vi "GetCalInfo.vi"(6 "Legacy (f)?":bool, 8 "error in (no error)":errorcluster) -> (0 "error out":errorcluster, 2 "CalInfo":T1)   [LabVIEW 2011]
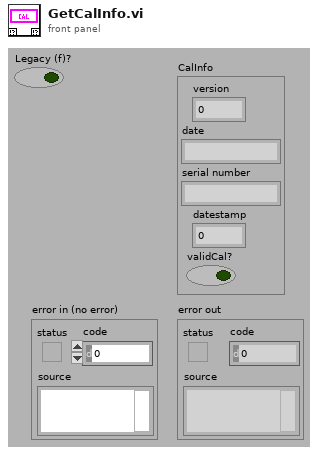
[diagram p1: front panel]
types:
  T1 = cluster{"version":u8, "date":string, "serial number":string, "datestamp":dbl, "validCal?":bool}
  T2 = cluster{"Command":string, "appended array":variant[]}
  T3 = cluster{"Command":string, "appended array":variant[]}[]
  T4 = cluster{"version":u8, "date":string, "serial number":string}
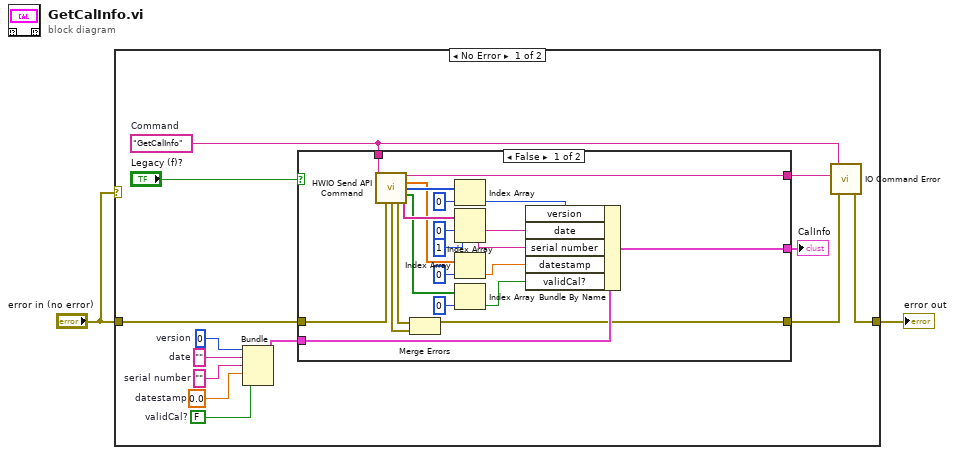
[diagram p0: block diagram]
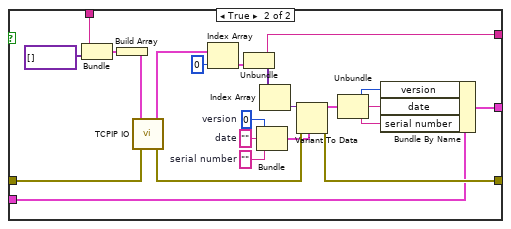
[diagram p2: hidden frame]
diagram:
  n1 = case shown="No Error" "error in (no error)" {
    tunnel: "error in (no error)" -> [w11 w61]
    tunnel: [w8 w61] -> w2
    frame No Error {
      w3 = FALSE  # validCal?
      w4 = 0.0  # datestamp
      w13 = u8 0  # version
      w15 = ""  # serial number
      w7 = "GetCalInfo"  # Command
      w14 = ""  # date
      n2 = Bundle("version"=w13, "date"=w14, "serial number"=w15, "datestamp"=w4, "validCal?"=w3) -> (w10:T1)  [unwired: 1 out]
      n3 = case shown="False" "Legacy (f)?" {
        tunnel: [w27 w42] -> w12
        tunnel: w11 -> [w37 w58]
        tunnel: w10 -> [w35 w43]
        tunnel: [w16 w56] -> w9
        tunnel: w7 -> [w36 w55]
        tunnel: [w26 w51] -> w6
        frame False {
          n4 = call "HWIO Send API Command.vi"("Action"=w36, "error in (no error)"=w37) -> ("Action out"=w26:string, "Double out"=w23:dbl[], "Integer out"=w31:i32[], "Boolean out"=w20:bool[], "HWError"=w17:errorcluster, "error out"=w18:errorcluster, "String out"=w30:string[])  [unwired: 6 in, 1 out]
          n5 = Merge Errors(w18, w17) -> (w16:errorcluster)
          n6 = Index Array(array=w31, index=0) -> (element=w28:i32)
          n7 = Index Array(array=w30, index #1=0 ("index"), index #2=1 ("index")) -> (element #1=w29:string, element #2=w25:string)
          n8 = Index Array(array=w23, index=0) -> (element=w22:dbl)
          n9 = Index Array(array=w20, index=0) -> (element=w19:bool)
          n10 = Bundle By Name(cluster=w35, "version"=w28, "date"=w29, "serial number"=w25, "datestamp"=w22, "validCal?"=w19) -> (w27:T1)
        }
        frame True {
          w46 = ""  # serial number
          w47 = ""  # date
          w45 = u8 0  # version
          n11 = Bundle("Command"=w55, "appended array"=variant[] []) -> (w60:T2)  [unwired: 1 out]
          n12 = Build Array(w60) -> (w54:T3)
          n13 = call "TCPIP IO.vi"("error in (no error)"=w58, "Commands"=w54) -> ("error out"=w57:errorcluster, "Responses"=w53:cluster{string, variant[]}[])  [unwired: 1 in, 3 out]
          n14 = Index Array(array=w53, index=0) -> (element=w52:cluster{string, variant[]})
          n15 = Unbundle(w52) -> (w51:string, w50:variant[])
          n16 = Bundle("version"=w45, "date"=w47, "serial number"=w46) -> (w44:T4)  [unwired: 1 out]
          n17 = Index Array(array=w50) -> (element=w49:variant)  [unwired: 1 in]
          n18 = Variant To Data(error in=w57, type=w44, Variant=w49) -> (data=w41:T4, error out=w56:errorcluster)
          n19 = Unbundle(w41) -> ("version"=w40:u8, "date"=w38:string, "serial number"=w39:string)
          n20 = Bundle By Name(cluster=w43, "version"=w40, "date"=w38, "serial number"=w39) -> (w42:T1)
        }
      }
      "CalInfo" <- w12
      n21 = call "IO Command Error.vi"("error in (no error)"=w9, "Command Returned (\"\")"=w6, "Command Sent (\"\")"=w7) -> ("error out"=w8:errorcluster)  [unwired: 4 out]
    }
    frame Error {
    }
  }
  "error out" <- w2
